vi "Read VI Refnum.vi"(8 "Error In":errorcluster, 11 "Model in":refnum<class "Model.lvclass">) -> (0 "Error Out":errorcluster, 2 "VI Refnum":refnum<vi>, 3 "Model out":refnum<class "Model.lvclass">)   [LabVIEW 2021, in "Model.lvclass"]
uses:
  Model.lvclass
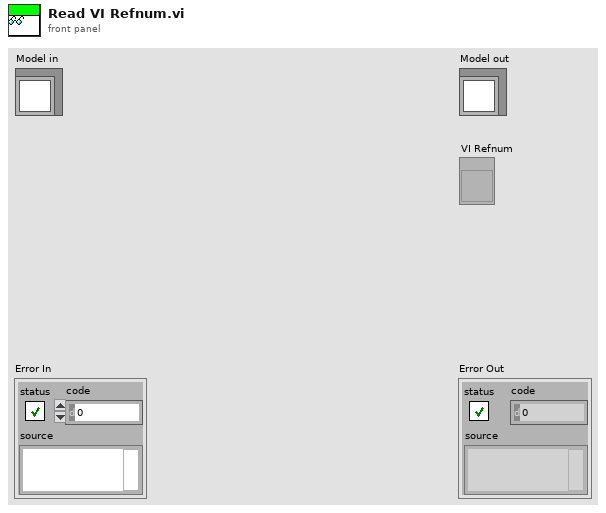
[diagram p1: front panel]
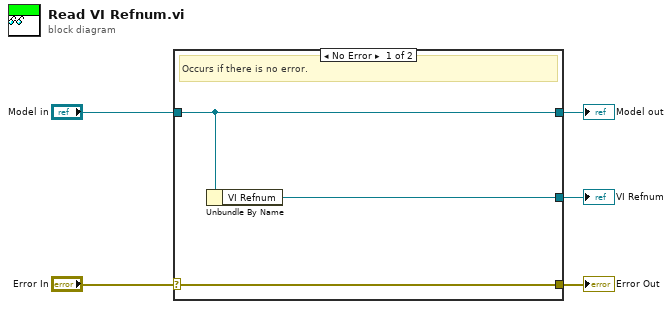
[diagram p0: block diagram]
diagram:
  n1 = case shown="No Error" "Error In" {
    selector: "Error In" -> [w8 w9]
    tunnel: [w8 w9] -> w4
    tunnel: [w7 w10] -> w2
    tunnel: "Model in" -> [w7 w10]
    tunnel: [w6 _] -> w1
    frame No Error {
      # "Occurs if there is no error."
      n2 = Unbundle By Name(w7) -> ("VI Refnum"=w6:refnum<vi>)
    }
    frame Error {
      # "Occurs if there is any error"
    }
  }
  "Error Out" <- w4
  "Model out" <- w2
  "VI Refnum" <- w1
